vi "Jenkins URL with Parameters Test.vi"() -> ()   [LabVIEW 2014]
uses:
  <vilib>/httpClient/LabVIEWHTTPClient.lvlib
  <vilib>/wsapi/NI_WebServices.lvlib
panel:
  out "error out 2":errorcluster
  out "body 2":string
  out "body":string
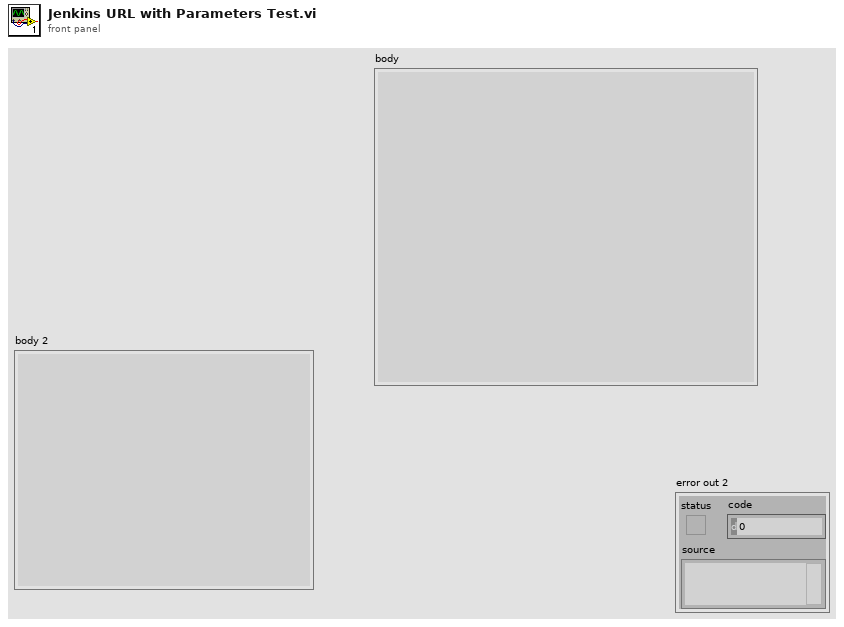
[diagram p1: front panel]
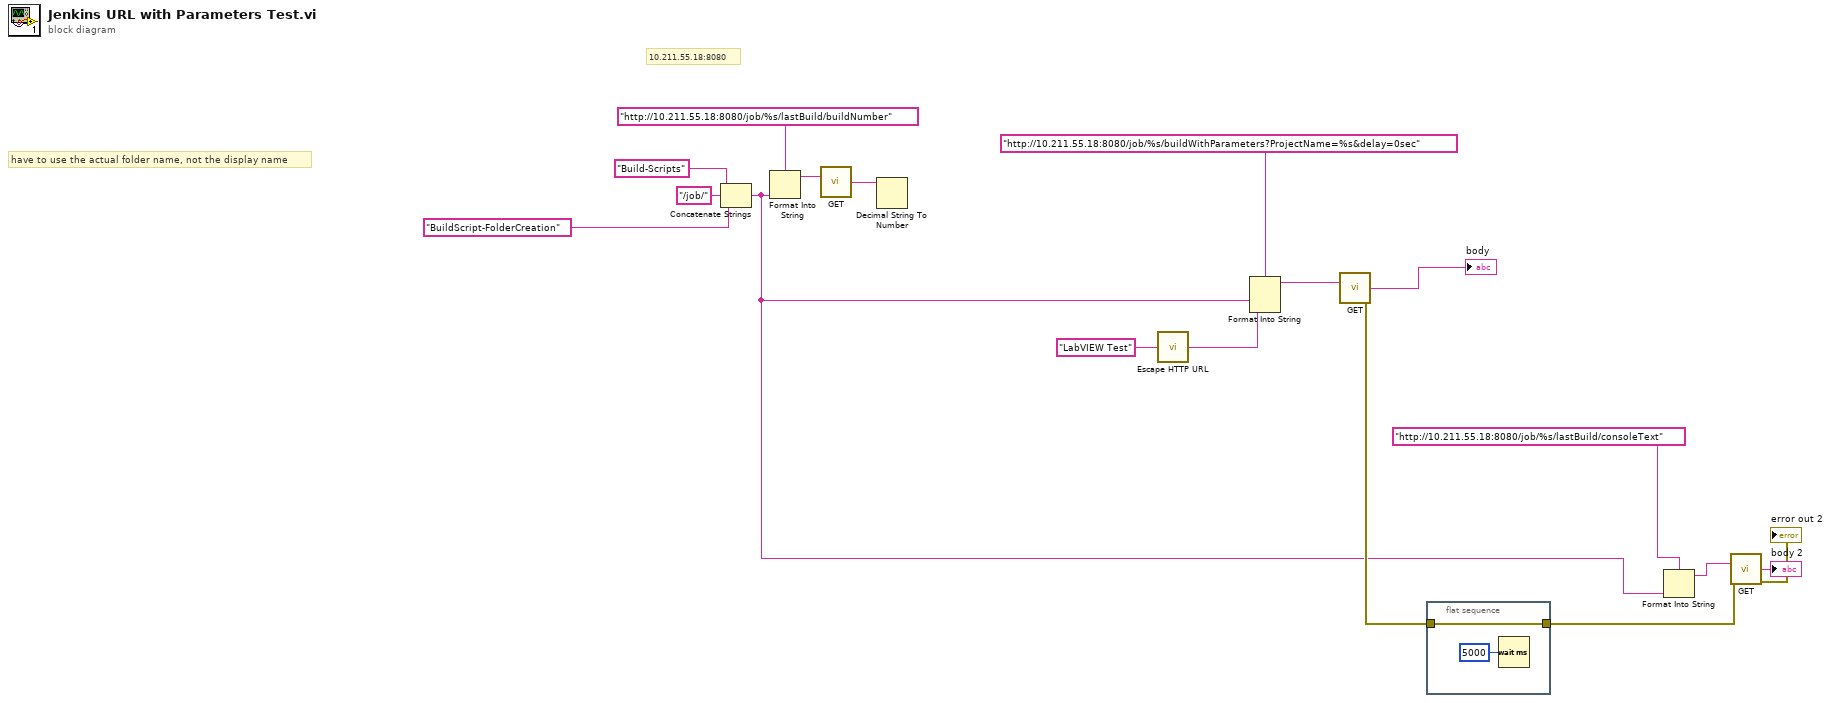
[diagram p0: block diagram]
diagram:
  # "10.211.55.18:8080"
  # "have to use the actual folder name, not the display name"
  n1 = Concatenate Strings("Build-Scripts" ("JSON"), "/job/" ("string"), "BuildScript-FolderCreation" ("JSON")) -> (w2:string)
  n2 = Format Into String(format string="http://10.211.55.18:8080/job/%s/lastBuild/buildNumber", w2) -> (resulting string=w18:string)  [unwired: 2 in, 1 out]
  n3 = call <vilib>:"GET.vi"("url"=w18) -> ("body"=w1:string)  [unwired: 11 in, 3 out]
  n4 = Decimal String To Number(string=w1) -> ()  [unwired: 2 in, 2 out]
  n5 = call <vilib>:"Escape HTTP URL.vi"("unescaped string in"="LabVIEW Test" ("JSON")) -> ("escaped string out"=w9:string)
  n6 = Format Into String(format string="http://10.211.55.18:8080/job/%s/buildWithParameters?ProjectName=%s&delay=0sec", w2, w9) -> (resulting string=w13:string)  [unwired: 2 in, 1 out]
  n7 = call <vilib>:"GET.vi"("url"=w13) -> ("body"=→"body":string, "error out"=w5:errorcluster)  [unwired: 11 in, 2 out]
  n8 = flat-sequence {
    tunnel: w5 -> [w20]
    tunnel: [w20] -> w4
    frame #0 {
      n9 = Wait (ms)(milliseconds to wait=u32 5000) -> ()  [unwired: 1 out]
    }
  }
  n10 = Format Into String(format string="http://10.211.55.18:8080/job/%s/lastBuild/consoleText", w2) -> (resulting string=w7:string)  [unwired: 2 in, 1 out]
  n11 = call <vilib>:"GET.vi"("url"=w7, "error in (no error)"=w4) -> ("body"=→"body 2":string, "error out"=→"error out 2":errorcluster)  [unwired: 10 in, 2 out]
